vi "BoilerMultiblock.vi"(7 "Boiler Build Properties":T2={"Water Tank (mB)"=0, "Steam Tank (mB)"=0, "Heated Coolant Tank (mB)"=0, "Coolant Tank (mB)"=0, "Maximum Boil Rate (mB/t)"=4, "Height (m)"=4, "Volume (m³)"=0, "Heat Capacity (J/K)"=0.0, "Pressure Dispersers"=4} {"Pressure Dispersers" min=4 max=18 step=1; "Height (m)" min=4 max=18 step=1; "Maximum Boil Rate (mB/t)" min=4 max=18 step=1}) -> ()   [LabVIEW 2026]
uses:
  Port Defs/Boiler Port States.ctl
  Boiler Build Properties.ctl
panel:
  out "Heated Coolant Tank (mB)":i64(slide) scale=-1.0..891000000.0
  out "Boiler Stats":dbl(graph)
  out "Temperature (K)":dbl
  in  "Biome Temperature":dbl=0.8
  out "Port States Out":T1
  in  "Port States In":T1
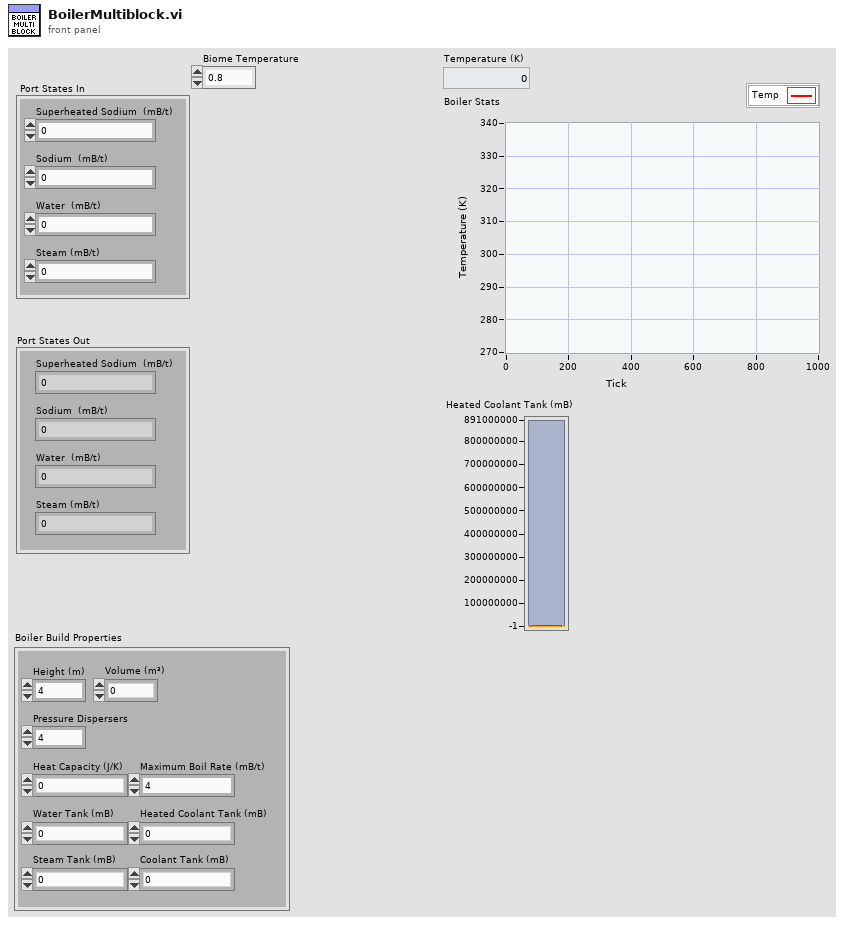
[diagram p1: front panel]
types:
  T1 = typedef "Boiler Port States.ctl" = cluster{"Superheated Sodium  (mB/t)":i64, "Sodium  (mB/t)":i64, "Water  (mB/t)":i64, "Steam (mB/t)":i64}
  T2 = typedef "Boiler Build Properties.ctl" = cluster{"Water Tank (mB)":i32, "Steam Tank (mB)":i32, "Heated Coolant Tank (mB)":i64, "Coolant Tank (mB)":i64, "Maximum Boil Rate (mB/t)":i32, "Height (m)":i32, "Volume (m³)":i32, "Heat Capacity (J/K)":dbl, "Pressure Dispersers":i32}
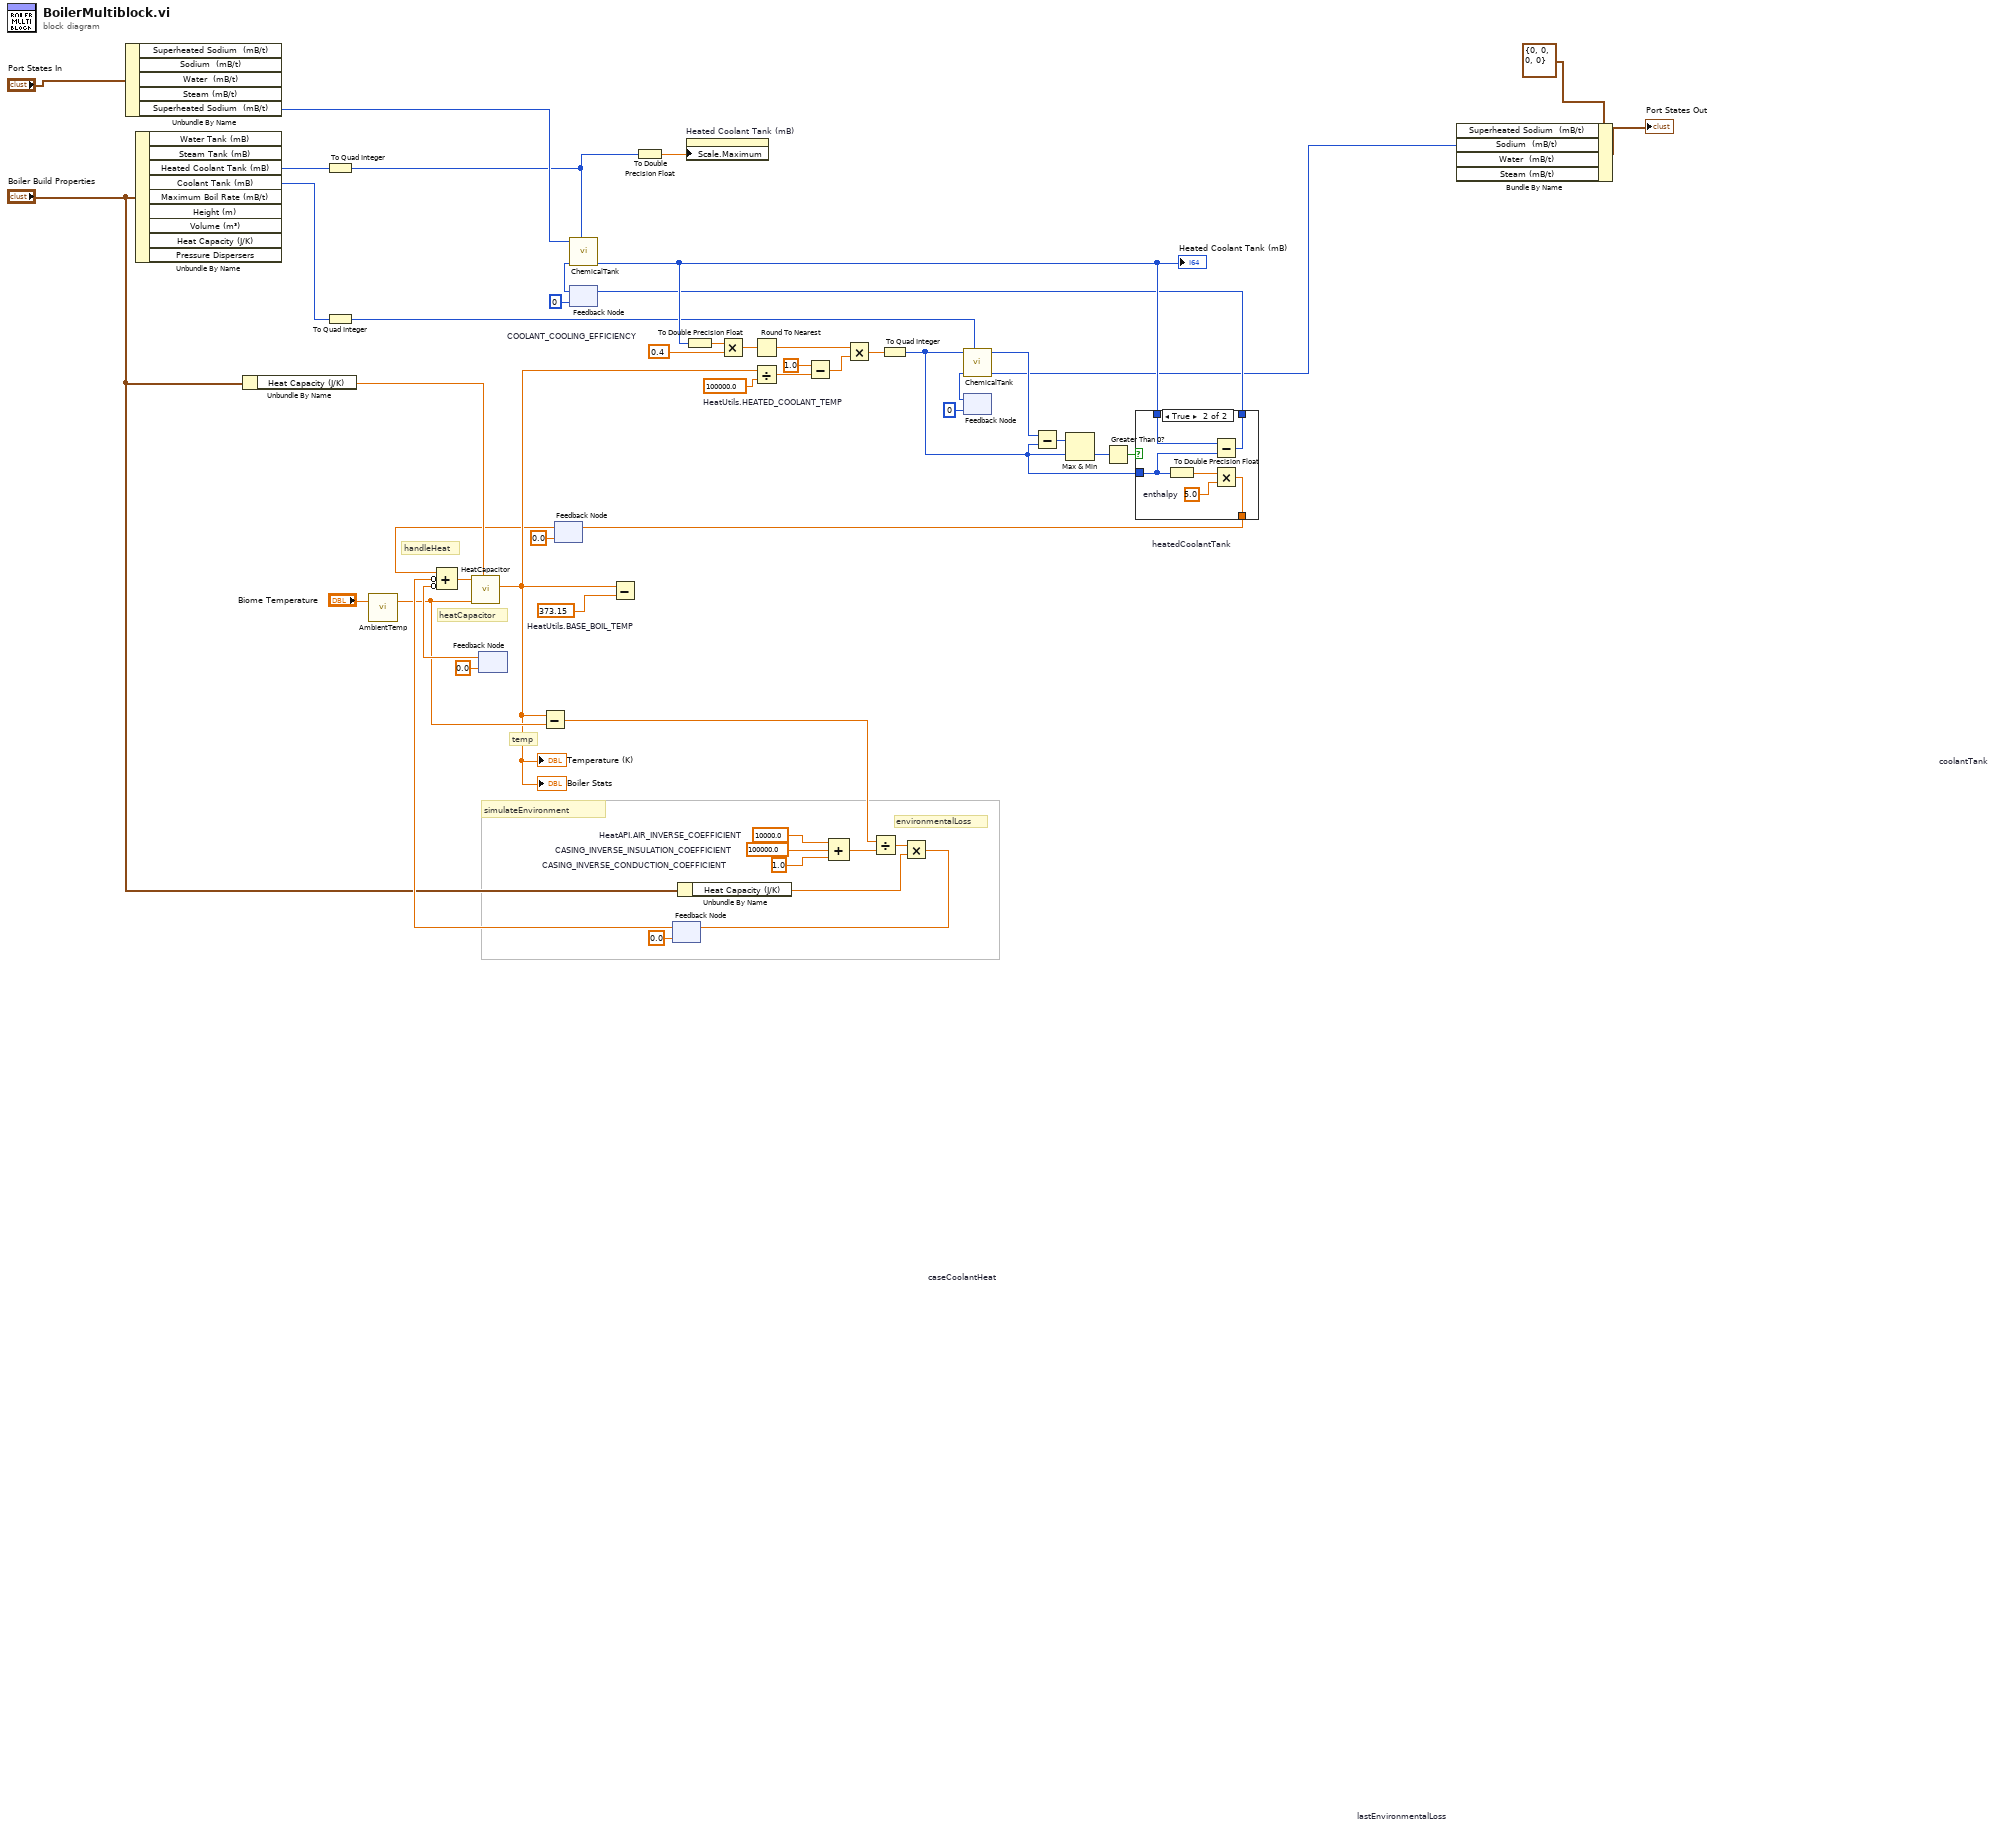
[diagram p0: block diagram]
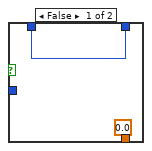
[diagram p2: hidden frame]
diagram:
  w22 = 100000.0  # HeatUtils.HEATED_COOLANT_TEMP
  w26 = 0.4  # COOLANT_COOLING_EFFICIENCY
  w45 = 373.15  # HeatUtils.BASE_BOIL_TEMP
  w48 = 1.0  # CASING_INVERSE_CONDUCTION_COEFFICIENT
  w49 = 100000.0  # CASING_INVERSE_INSULATION_COEFFICIENT
  w50 = 10000.0  # HeatAPI.AIR_INVERSE_COEFFICIENT
  # "simulateEnvironment"
  # "handleHeat"
  # "temp"
  # "heatCapacitor"
  # "environmentalLoss"
  n1 = Unbundle By Name("Port States In") -> ("Superheated Sodium  (mB/t)"=w29:i64)  [unwired: 4 out]
  n2 = Unbundle By Name("Boiler Build Properties") -> ("Heated Coolant Tank (mB)"=w31:i64, "Coolant Tank (mB)"=w16:i64)  [unwired: 7 out]
  n3 = Unbundle By Name("Boiler Build Properties") -> ("Heat Capacity (J/K)"=w35:dbl)
  n4 = To Quad Integer(1:w31) -> (0:w27:i64)
  n5 = To Quad Integer(1:w16) -> (0:w15:i64)
  n6 = call "AmbientTemp.vi"("Biome Temperature"="Biome Temperature") -> ("Biome Ambient Temp (K)"=w37:dbl)  [unwired: 18 in]
  n7 = feedback #1 "caseCoolantHeat"(0.0) -> (w42:dbl)
  n8 = feedback-in #1() -> ()  [unwired: 1 out]
  n9 = feedback #2(0.0) -> (w9:dbl)
  n10 = feedback #3 "heatedCoolantTank"(i64 0 ("Fill (mB)")) -> (w33:i64)
  n11 = call "ChemicalTank.vi"("Capacity (mB)"=w27, "Last Fill (mB)"=w33, "Transfer (mB)"=w29) -> ("Fill (mB)"=w52:i64)  [unwired: 2 in, 3 out]
  "Heated Coolant Tank (mB)" <- w52
  n12 = To Double Precision Float(number=w27) -> (double precision float=w28:dbl)
  n13 = feedback #4 "lastEnvironmentalLoss"(0.0) -> (w38:dbl)
  n14 = Compound Arithmetic op=ADD(w9, invert w38, invert w42) -> (w44:dbl)
  n15 = call "HeatCapacitor.vi"("Capacity (J/K)"=w35, "Ambient Temperature (K)"=w37, "Transfer (J)"=w44) -> ("Temperature (K)"=w23:dbl)  [unwired: 7 in, 1 out]
  "Temperature (K)" <- w23
  "Boiler Stats" <- w23
  n16 = Subtract(x=w23, y=w37) -> (x-y=w41:dbl)
  n17 = Subtract(x=w23, y=w45) -> ()  [unwired: 1 out]
  n18 = Unbundle By Name("Boiler Build Properties") -> ("Heat Capacity (J/K)"=w36:dbl)
  n19 = property on="Heated Coolant Tank (mB)" class="Slide (strict)"("Scale.Maximum"=w28) -> ()  [unwired: 2 in, 2 out]
  n20 = To Double Precision Float(number=w52) -> (double precision float=w25:dbl)
  n21 = Multiply(x=w25, y=w26) -> (x*y=w24:dbl)
  n22 = Round To Nearest(number=w24) -> (nearest integer value=w19:dbl)
  n23 = Divide(x=w23, y=w22) -> (x/y=w20:dbl)
  n24 = Subtract(x=1.0, y=w20) -> (x-y=w18:dbl)
  n25 = Compound Arithmetic op=unknown(w50, w49, w48) -> (w47:dbl)
  n26 = Multiply(x=w19, y=w18) -> (x*y=w17:dbl)
  n27 = Divide(x=w41, y=w47) -> (x/y=w46:dbl)
  n28 = To Quad Integer(1:w17) -> (0:w4:i64)
  n29 = Multiply(x=w46, y=w36) -> (x*y=w39:dbl)
  n30 = feedback-in #4(w39) -> ()
  n31 = feedback #5 "coolantTank"(i64 0 ("Fill (mB)")) -> (w5:i64)
  n32 = call "ChemicalTank.vi"("Capacity (mB)"=w15, "Last Fill (mB)"=w5, "Transfer (mB)"=w4) -> ("Fill (mB)"=w1:i64, "Overflow (mB)"=w14:i64)  [unwired: 2 in, 2 out]
  n33 = feedback-in #5() -> ()  [unwired: 1 out]
  n34 = Subtract(x=w14, y=w4) -> (x-y=w13:i64)
  n35 = Max & Min(x=w13, y=w4) -> (min(x,y)=w12:i64)  [unwired: 1 out]
  n36 = Greater Than 0?(x=w12) -> (x > 0?=w11:bool)
  n37 = case shown="True" w11 {
    tunnel: w4 -> [_ w56]
    tunnel: [0.0 w58] -> w10
    tunnel: w52 -> [w54 w57]
    tunnel: [w54 w55] -> w7
    frame False {
    }
    frame True {
      w60 = 5.0  # enthalpy
      n38 = To Double Precision Float(number=w56) -> (double precision float=w59:dbl)
      n39 = Subtract(x=w57, y=w56) -> (x-y=w55:i64)
      n40 = Multiply(x=w59, y=w60) -> (x*y=w58:dbl)
    }
  }
  n41 = feedback-in #2(w10) -> ()
  n42 = feedback-in #3(w7) -> ()
  n43 = Bundle By Name(cluster=T1 {"Superheated Sodium  (mB/t)"=0, "Sodium  (mB/t)"=0, "Water  (mB/t)"=0, "Steam (mB/t)"=0} ("Port States Out"), "Sodium  (mB/t)"=w1) -> (→"Port States Out":T1)  [unwired: 3 in]
